vi "test-create-path-trajectory.vi"() -> ()   [LabVIEW 2019]
uses:
  <vilib>/Rock Robotics/WPI/ThirdParty/MJansen/PathPlanner/PathPlanner24.lvlib
  <vilib>/Rock Robotics/WPI/ThirdParty/JAS_Junk/TrajLib/Trajectory_Library.lvlib
  <vilib>/Rock Robotics/WPI/ThirdParty/JAS_Junk/TrajLib/TypeDef/ROTATION2D.ctl
  <vilib>/Rock Robotics/WPI/ThirdParty/JAS_Junk/TrajLib/TypeDef/TRANSLATION2D.ctl
  <vilib>/Rock Robotics/WPI/ThirdParty/JAS_Junk/TrajLib/TypeDef/POSE2D.ctl
  <vilib>/Rock Robotics/WPI/ThirdParty/JAS_Junk/TrajLib/TypeDef/TRAJ_STATE.ctl
  <vilib>/Rock Robotics/WPI/ThirdParty/MJansen/PathPlanner/TypeDef/PathPlannerTrajectoryState.ctl
  <vilib>/Rock Robotics/WPI/ThirdParty/MJansen/PathPlanner/TypeDef/PathPlannerTrajectory.ctl
  <vilib>/Rock Robotics/WPI/ThirdParty/MJansen/PathPlanner/TypeDef/PathPlannerPathConstraints.ctl
  <vilib>/Rock Robotics/WPI/ThirdParty/JAS_Junk/TrajLib/TypeDef/CHASSIS_SPEEDS.ctl
  <vilib>/Rock Robotics/WPI/ThirdParty/MJansen/PathPlanner/TypeDef/PathPlannerGoalEndState.ctl
  <vilib>/Rock Robotics/WPI/ThirdParty/MJansen/PathPlanner/TypeDef/PathPlannerRotationTarget.ctl
  <vilib>/Rock Robotics/WPI/ThirdParty/MJansen/PathPlanner/TypeDef/PathPlannerConstraintsZone.ctl
  <vilib>/Rock Robotics/WPI/ThirdParty/MJansen/PathPlanner/TypeDef/PathPlannerEventMarker.ctl
  <vilib>/Rock Robotics/WPI/ThirdParty/MJansen/PathPlanner/TypeDef/PathPlannerPathPoint.ctl
  <vilib>/Rock Robotics/WPI/ThirdParty/MJansen/PathPlanner/TypeDef/PathPlannerPath.ctl
  <vilib>/Rock Robotics/WPI/ThirdParty/MJansen/PathPlanner/ENum/PathPlanner_CommandUtilType_ENUM.ctl
  <vilib>/Rock Robotics/WPI/ThirdParty/MJansen/PathPlanner/TypeDef/PathPlannerCommandUtil.ctl
  <vilib>/Rock Robotics/WPI/ThirdParty/MJansen/PathPlanner/TypeDef/PathPlannerWaypoint.ctl
  <vilib>/Rock Robotics/WPI/ThirdParty/MJansen/PathPlanner/TypeDef/PathPlannerPointTowardsZone.ctl
  <vilib>/Rock Robotics/WPI/ThirdParty/MJansen/PathPlanner/TypeDef/PathPlannerIdealStartingState.ctl
panel:
  in  "Tab Control":T1(tab)
  in  "Position 1":T2={"TRANSLATION"={"X"=1.0, "Y"=1.0}, "ROTATION"={"VALUE"=0.0, "COS"=1.0, "SIN"=0.0}} {"ROTATION"."SIN" format="%13.4f"; "ROTATION"."COS" format="%13.4f"; "ROTATION"."VALUE" format="%13.4f"; "TRANSLATION"."Y" format="%14.3f"; "TRANSLATION"."X" format="%14.3f"}
  in  "Position 2":T2={"TRANSLATION"={"X"=2.0, "Y"=1.0}, "ROTATION"={"VALUE"=0.0, "COS"=1.0, "SIN"=0.0}} {"ROTATION"."SIN" format="%13.4f"; "ROTATION"."COS" format="%13.4f"; "ROTATION"."VALUE" format="%13.4f"; "TRANSLATION"."Y" format="%14.3f"; "TRANSLATION"."X" format="%14.3f"}
  in  "Position 3":T2={"TRANSLATION"={"X"=3.0, "Y"=1.0}, "ROTATION"={"VALUE"=0.0, "COS"=1.0, "SIN"=0.0}} {"ROTATION"."SIN" format="%13.4f"; "ROTATION"."COS" format="%13.4f"; "ROTATION"."VALUE" format="%13.4f"; "TRANSLATION"."Y" format="%14.3f"; "TRANSLATION"."X" format="%14.3f"}
  in  "Position 4":T2={"TRANSLATION"={"X"=4.0, "Y"=1.0}, "ROTATION"={"VALUE"=0.0, "COS"=1.0, "SIN"=0.0}} {"ROTATION"."SIN" format="%13.4f"; "ROTATION"."COS" format="%13.4f"; "ROTATION"."VALUE" format="%13.4f"; "TRANSLATION"."Y" format="%14.3f"; "TRANSLATION"."X" format="%14.3f"}
  in  "stop":bool
  in  "StartingSpeeds":T5 {"vOmega" format="%10.3f"; "vY" format="%10.3f"; "vX" format="%10.3f"}
  out "Error":bool
  out "Error 2":bool
  out "PathPlannerConstraints":T6={"MaxVelocityMps;"=0.0, "MaxAccelerationMpsSq;"=0.0, "MaxAngularVelRadPsEc;"=0.0, "MaxAngularAccRadPSecSq"=0.0, "Exists"=FALSE, "Unlimited"=FALSE, "NominalVoltageVolts"=12.0}
  out "GoalEndState":T7={"VelocityMPS"=0.0, "Rotation"={"VALUE"=0.0, "COS"=1.0, "SIN"=0.0}} {"Rotation"."SIN" format="%13.4f"; "Rotation"."COS" format="%13.4f"; "Rotation"."VALUE" format="%13.4f"}
  out "PathPlannerPath":T8={"Reversed"=FALSE, "RotationTargets"=[], "ConstraintZones"=[], "EventMarkers"=[], "GlobalConstraints"={"MaxVelocityMps;"=0.0, "MaxAccelerationMpsSq;"=0.0, "MaxAngularVelRadPsEc;"=0.0, "MaxAngularAccRadPSecSq"=0.0, "Exists"=FALSE, "Unlimited"=FALSE, "NominalVoltageVolts"=1.0}, "GoalEndState"={"VelocityMPS"=0.0, "Rotation"={"VALUE"=0.0, "COS"=1.0, "SIN"=0.0}}, "AllPoints"=[], "Name"="", "Waypoints"=[], "PointTowardsZones"=[], "IdealStartingState"={"VelocityMPS"=0.0, "Rotation"={"VALUE"=0.0, "COS"=1.0, "SIN"=0.0}}, "IsChoreoPath"=FALSE, "PreventFlipping"=FALSE} {"IdealStartingState"."Rotation"."SIN" format="%13.4f"; "IdealStartingState"."Rotation"."COS" format="%13.4f"; "IdealStartingState"."Rotation"."VALUE" format="%13.4f"; "PointTowardsZones"."TargetPosition"."Y" format="%14.3f"; "PointTowardsZones"."TargetPosition"."X" format="%14.3f"; "PointTowardsZones"."RotationOffset"."SIN" format="%13.4f"; "PointTowardsZones"."RotationOffset"."COS" format="%13.4f"; "PointTowardsZones"."RotationOffset"."VALUE" format="%13.4f"; "Waypoints"."nextControl"."Y" format="%14.3f"; "Waypoints"."nextControl"."X" format="%14.3f"; "Waypoints"."anchor"."Y" format="%14.3f"; "Waypoints"."anchor"."X" format="%14.3f"; "Waypoints"."prevControl"."Y" format="%14.3f"; "Waypoints"."prevControl"."X" format="%14.3f"; "AllPoints"."RotationTarget"."rotation"."SIN" format="%13.4f"; "AllPoints"."RotationTarget"."rotation"."COS" format="%13.4f"; "AllPoints"."RotationTarget"."rotation"."VALUE" format="%13.4f"; "AllPoints"."Position"."Y" format="%14.3f"; "AllPoints"."Position"."X" format="%14.3f"; "GoalEndState"."Rotation"."SIN" format="%13.4f"; "GoalEndState"."Rotation"."COS" format="%13.4f"; "GoalEndState"."Rotation"."VALUE" format="%13.4f"; "RotationTargets"."rotation"."SIN" format="%13.4f"; "RotationTargets"."rotation"."COS" format="%13.4f"; "RotationTargets"."rotation"."VALUE" format="%13.4f"}
  out "PathPlannerTrajectory":T18 {"States"."TargetHolonomicRotation"."SIN" format="%13.4f"; "States"."TargetHolonomicRotation"."COS" format="%13.4f"; "States"."TargetHolonomicRotation"."VALUE" format="%13.4f"; "States"."Heading"."SIN" format="%13.4f"; "States"."Heading"."COS" format="%13.4f"; "States"."Heading"."VALUE" format="%13.4f"; "States"."PositionMeters"."Y" format="%14.3f"; "States"."PositionMeters"."X" format="%14.3f"}
  out "outPathPlannerStates":T19[](array[typedef]) {"TargetHolonomicRotation"."SIN" format="%13.4f"; "TargetHolonomicRotation"."COS" format="%13.4f"; "TargetHolonomicRotation"."VALUE" format="%13.4f"; "Heading"."SIN" format="%13.4f"; "Heading"."COS" format="%13.4f"; "Heading"."VALUE" format="%13.4f"; "PositionMeters"."Y" format="%14.3f"; "PositionMeters"."X" format="%14.3f"}
  in  "Down Button":bool
  in  "Up Button":bool
  in  "index":i32 step=20
  out "LabVIEWStateCount":i32
  out "LabVIEWStates":T20[](array[typedef]) {"POSE"."ROTATION"."SIN" format="%13.4f"; "POSE"."ROTATION"."COS" format="%13.4f"; "POSE"."ROTATION"."VALUE" format="%13.4f"; "POSE"."TRANSLATION"."Y" format="%14.3f"; "POSE"."TRANSLATION"."X" format="%14.3f"}
  out "XY SPLINE":cluster{dbl[], dbl[]}[](graph)
  out "XY Graph":cluster{dbl[], dbl[]}[](graph)
  out "Sample Graph":dbl[][](graph)
  out "LabVIEW Time Plot":cluster{dbl[], dbl[]}[](graph)
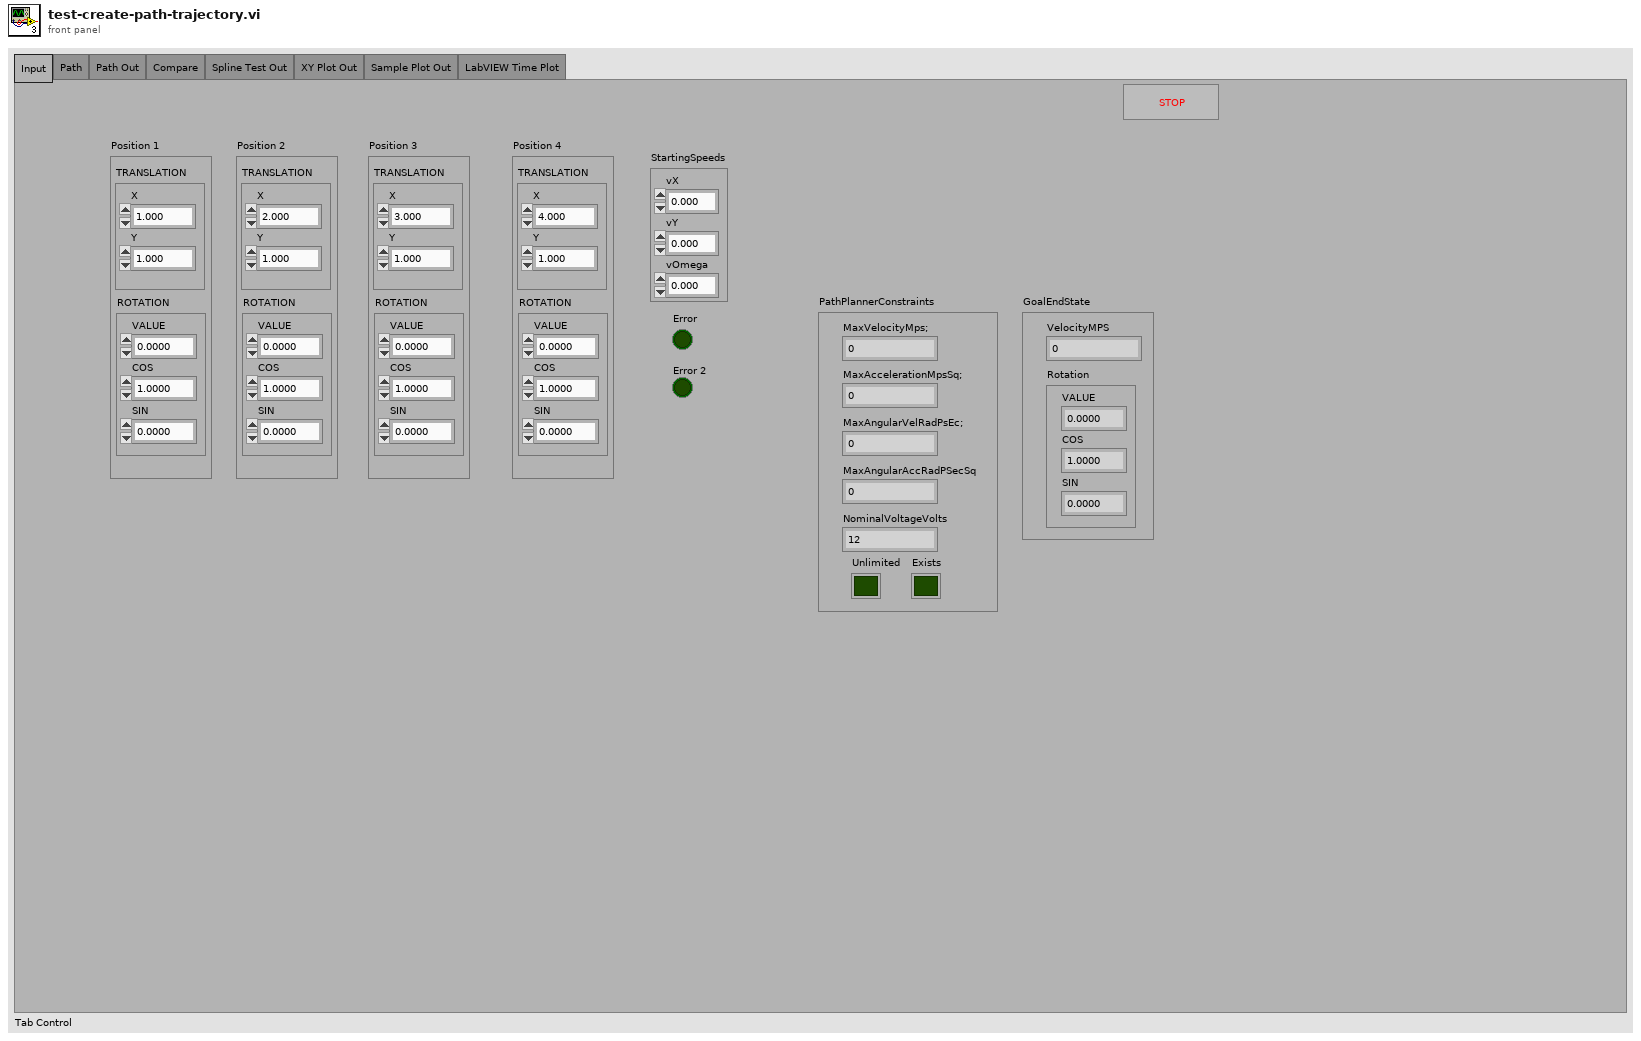
[diagram p1: front panel]
types:
  T1 = enum32{"Input", "Path", "Path Out", "Compare", "Spline Test Out", "XY Plot Out", "Sample Plot Out", "LabVIEW Time Plot"}
  T2 = typedef "Trajectory_Library.lvlib/POSE2D.ctl" = cluster{"TRANSLATION":T3, "ROTATION":T4}
  T3 = typedef "Trajectory_Library.lvlib/TRANSLATION2D.ctl" = cluster{"X":dbl, "Y":dbl}
  T4 = typedef "Trajectory_Library.lvlib/ROTATION2D.ctl" = cluster{"VALUE":dbl, "COS":dbl, "SIN":dbl}
  T5 = typedef "Trajectory_Library.lvlib/CHASSIS_SPEEDS.ctl" = cluster{"vX":dbl, "vY":dbl, "vOmega":dbl}
  T6 = typedef "PathPlanner24.lvlib/PathPlannerPathConstraints.ctl" = cluster{"MaxVelocityMps;":dbl, "MaxAccelerationMpsSq;":dbl, "MaxAngularVelRadPsEc;":dbl, "MaxAngularAccRadPSecSq":dbl, "Exists":bool, "Unlimited":bool, "NominalVoltageVolts":dbl}
  T7 = typedef "PathPlanner24.lvlib/PathPlannerGoalEndState.ctl" = cluster{"VelocityMPS":dbl, "Rotation":T4}
  T8 = typedef "PathPlanner24.lvlib/PathPlannerPath.ctl" = cluster{"Reversed":bool, "RotationTargets":T9[], "ConstraintZones":T10[], "EventMarkers":T11[], "GlobalConstraints":T6, "GoalEndState":T7, "AllPoints":T14[], "Name":string, "Waypoints":T15[], "PointTowardsZones":T16[], "IdealStartingState":T17, "IsChoreoPath":bool, "PreventFlipping":bool}
  T9 = typedef "PathPlanner24.lvlib/PathPlannerRotationTarget.ctl" = cluster{"position":dbl, "rotation":T4, "Exists":bool}
  T10 = typedef "PathPlanner24.lvlib/PathPlannerConstraintsZone.ctl" = cluster{"minPosition":dbl, "maxPosition":dbl, "Constraints":T6, "Present":bool}
  T11 = typedef "PathPlanner24.lvlib/PathPlannerEventMarker.ctl" = cluster{"Position":dbl, "Command":T12, "TriggerName":string, "EndPosition":dbl}
  T12 = typedef "PathPlanner24.lvlib/PathPlannerCommandUtil.ctl" = cluster{"waitTime":dbl, "name":string, "pathName":string, "commands":cluster{"type":T13, "waitTime":dbl, "name":string, "pathName":string}[], "type":T13}
  T13 = typedef "PathPlanner24.lvlib/PathPlanner_CommandUtilType_ENUM.ctl" = enum16{"Unknown", "Wait", "Named", "Path", "Sequential", "Parallel", "Race", "Deadline"}
  T14 = typedef "PathPlanner24.lvlib/PathPlannerPathPoint.ctl" = cluster{"Position":T3, "DistAlongPath":dbl, "MaxV":dbl, "Constraints":T6, "RotationTarget":T9, "WaypointRelativePos":dbl}
  T15 = typedef "PathPlanner24.lvlib/PathPlannerWaypoint.ctl" = cluster{"prevControl":T3, "anchor":T3, "nextControl":T3, "PrevExists":bool, "NextExists":bool}
  T16 = typedef "PathPlanner24.lvlib/PathPlannerPointTowardsZone.ctl" = cluster{"RotationOffset":T4, "Name":string, "TargetPosition":T3, "MinPosition":dbl, "MaxPosition":dbl}
  T17 = typedef "PathPlanner24.lvlib/PathPlannerIdealStartingState.ctl" = cluster{"VelocityMPS":dbl, "Rotation":T4}
  T18 = typedef "PathPlanner24.lvlib/PathPlannerTrajectory.ctl" = cluster{"States":T19[]}
  T19 = typedef "PathPlanner24.lvlib/PathPlannerTrajectoryState.ctl" = cluster{"TimeSeconds":dbl, "VelocityMPS":dbl, "AccerationMpsSq":dbl, "HeadingAngularVelRadPerSec":dbl, "PositionMeters":T3, "Heading":T4, "TargetHolonomicRotation":T4, "CurvatureRadPerMeter":dbl, "PathPlannerConstraints":T6, "DeltaPos":dbl}
  T20 = typedef "Trajectory_Library.lvlib/TRAJ_STATE.ctl" = cluster{"TimeSeconds":dbl, "Velocity":dbl, "Acceleration":dbl, "POSE":T2, "Curvature":dbl}
  T21 = typedef "Trajectory_Library.lvlib/TRAJECTORY.ctl" = cluster{"TotalTImeSecs":dbl, "States":T20[]}
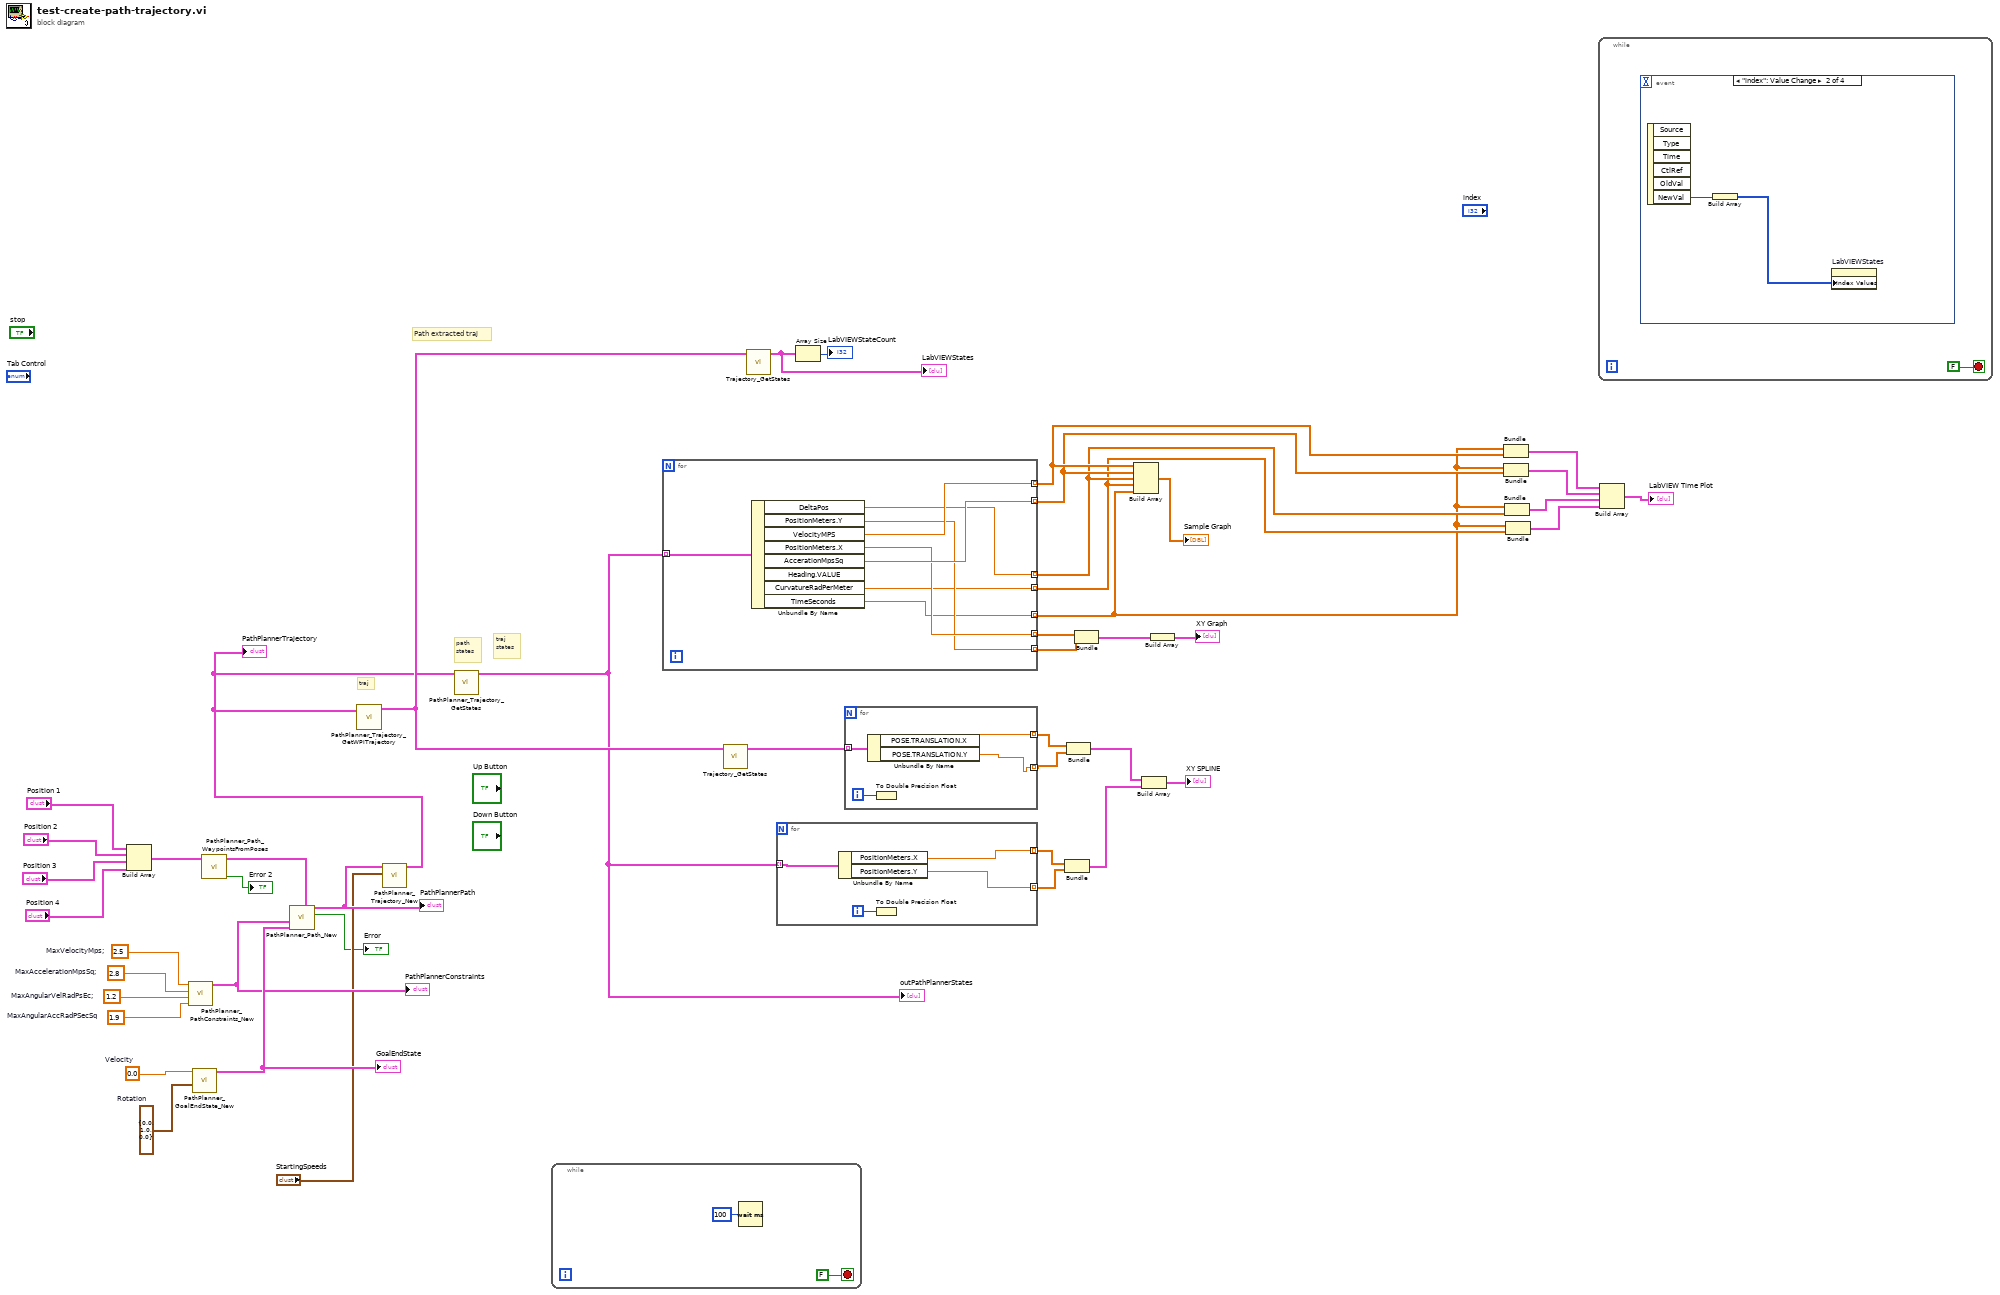
[diagram p0: block diagram]
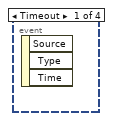
[diagram p2: hidden frame]
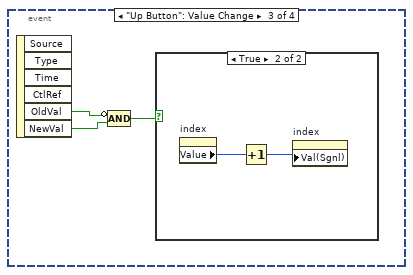
[diagram p3: hidden frame]
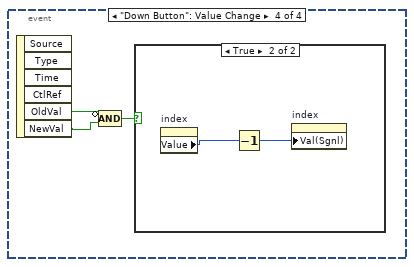
[diagram p5: hidden frame]
diagram:
  w6 = 0.0  # Velocity
  w7 = T4 {"VALUE"=0.0, "COS"=1.0, "SIN"=0.0}  # Rotation
  w9 = 2.5  # MaxVelocityMps;
  w10 = 2.8  # MaxAccelerationMpsSq;
  w11 = 1.2  # MaxAngularVelRadPsEc;
  w8 = 1.9  # MaxAngularAccRadPSecSq
  # "Path extracted traj"
  # "traj"
  # "traj\nstates"
  # "path\nstates"
  n1 = Build Array("Position 1", "Position 2", "Position 3", "Position 4") -> (w15:T2[])
  n2 = call <vilib>:"PathPlanner_PathConstraints_New.vi"("MaxAngularAccRadPSecSq"=w8, "MaxAngularVelRadPsEc;"=w11, "MaxAccelerationMpsSq;"=w10, "MaxVelocityMps;"=w9) -> ("PathPlannerConstraints"=w12:T6)  [unwired: 7 in]
  "PathPlannerConstraints" <- w12
  n3 = call <vilib>:"PathPlanner_GoalEndState_New.vi"("Rotation"=w7, "VelocityMPS"=w6) -> ("GoalEndState"=w13:T7)  [unwired: 9 in]
  "GoalEndState" <- w13
  n4 = call <vilib>:"PathPlanner_Path_WaypointsFromPoses.vi"("Poses"=w15) -> ("Error"=→"Error 2":bool, "Waypoints"=w14:T15[])  [unwired: 9 in]
  n5 = call <vilib>:"PathPlanner_Path_New.vi"("Waypoints"=w14, "GoalEndState"=w13, "GlobalConstraints"=w12) -> ("Error"=→"Error":bool, "PathPlannerPath"=w5:T8)  [unwired: 7 in]
  "PathPlannerPath" <- w5
  n6 = call <vilib>:"PathPlanner_Trajectory_New.vi"("StartingSpeeds"="StartingSpeeds", "Path"=w5) -> ("PathPlannerTrajectory"=w4:T18)  [unwired: 8 in, 1 out]
  "PathPlannerTrajectory" <- w4
  n7 = call <vilib>:"PathPlanner_Trajectory_GetWPITrajectory.vi"("PathPlannerTrajectory"=w4) -> ("WPI TRAJECTORY"=w33:T21)  [unwired: 9 in, 1 out]
  n8 = call <vilib>:"PathPlanner_Trajectory_GetStates.vi"("PathPlannerTrajectory"=w4) -> ("PathPlannerStates"=w30:T19[])  [unwired: 10 in]
  "outPathPlannerStates" <- w30
  n9 = while {
    stop <- FALSE stop-if-true
    n10 = Wait (ms)(milliseconds to wait=u32 100) -> ()  [unwired: 1 out]
  }
  n11 = for {
    tunnel: [w56] -> w28 mode=indexing
    tunnel: [w55] -> w27 mode=indexing
    tunnel: [w50] -> w26 mode=indexing
    tunnel: [w54] -> w45 mode=indexing
    tunnel: [w53] -> w44 mode=indexing
    tunnel: w30 -> [w52] mode=indexing
    tunnel: [w51] -> w25 mode=indexing
    tunnel: [w49] -> w20 mode=indexing
    n12 = Unbundle By Name(w52) -> ("DeltaPos"=w50:dbl, "PositionMeters.Y"=w53:dbl, "VelocityMPS"=w56:dbl, "PositionMeters.X"=w54:dbl, "AccerationMpsSq"=w55:dbl, "CurvatureRadPerMeter"=w51:dbl, "TimeSeconds"=w49:dbl)  [unwired: 1 out]
  }
  n13 = call <vilib>:"Trajectory_GetStates.vi"("TRAJECTORY"=w33) -> ("States"=w34:T20[])  [unwired: 10 in]
  n14 = call <vilib>:"Trajectory_GetStates.vi"("TRAJECTORY"=w33) -> ("States"=w31:T20[])  [unwired: 10 in]
  "LabVIEWStates" <- w31
  n15 = for {
    tunnel: [w59] -> w39 mode=indexing
    tunnel: w30 -> [w58] mode=indexing
    tunnel: [w57] -> w38 mode=indexing
    i -> [w60]
    n16 = Unbundle By Name(w58) -> ("PositionMeters.X"=w59:dbl, "PositionMeters.Y"=w57:dbl)
    n17 = To Double Precision Float(number=w60) -> ()  [unwired: 1 out]
  }
  n18 = Array Size(array=w31) -> (size(s)=→"LabVIEWStateCount":i32)
  n19 = for {
    tunnel: [w63] -> w41 mode=indexing
    tunnel: [w62] -> w40 mode=indexing
    tunnel: w34 -> [w61] mode=indexing
    i -> [w64]
    n20 = Unbundle By Name(w61) -> ("POSE.TRANSLATION.X"=w63:dbl, "POSE.TRANSLATION.Y"=w62:dbl)
    n21 = To Double Precision Float(number=w64) -> ()  [unwired: 1 out]
  }
  n22 = Bundle(w39, w38) -> (w36:cluster{dbl[], dbl[]})  [unwired: 1 in]
  n23 = Bundle(w41, w40) -> (w37:cluster{dbl[], dbl[]})  [unwired: 1 in]
  n24 = Bundle(w45, w44) -> (w43:cluster{dbl[], dbl[]})  [unwired: 1 in]
  n25 = Build Array(w28, w27, w26, w25, w20) -> (→"Sample Graph":dbl[][])
  n26 = Build Array(w37, w36) -> (→"XY SPLINE":cluster{dbl[], dbl[]}[])
  n27 = Build Array(w43) -> (→"XY Graph":cluster{dbl[], dbl[]}[])
  n28 = Bundle(w20, w28) -> (w24:cluster{dbl[], dbl[]})  [unwired: 1 in]
  n29 = Bundle(w20, w27) -> (w23:cluster{dbl[], dbl[]})  [unwired: 1 in]
  n30 = Bundle(w20, w26) -> (w22:cluster{dbl[], dbl[]})  [unwired: 1 in]
  n31 = Bundle(w20, w25) -> (w21:cluster{dbl[], dbl[]})  [unwired: 1 in]
  n32 = while {
    stop <- FALSE stop-if-true
    n33 = event shown="[1] \"index\": Value Change" {
      selector: _ -> [_ _ _ _]
      dyn-events: _ -> [_ _ _ _]
      timeout: _ -> [_ _ _ _]
      event Timeout {
        n34 = event-data() -> ()  [unwired: 1 in, 3 out]
      }
      event "index": Value Change {
        n35 = event-data() -> ("NewVal"=w67:i32)  [unwired: 1 in, 5 out]
        n36 = Build Array(w67) -> (w66:i32[])
        n37 = property on="LabVIEWStates" class="Arr (strict)"("Index Values"=w66) -> ()  [unwired: 2 in, 2 out]
      }
      event "Up Button": Value Change {
        n38 = event-data() -> ("OldVal"=w70:bool, "NewVal"=w69:bool)  [unwired: 1 in, 4 out]
        n39 = Compound Arithmetic op=AND(invert w70, w69) -> (w68:bool)
        n40 = case shown="True" w68 {
          frame False {
          }
          frame True {
            n41 = property on="index" class="DigNum (strict)"() -> ("Value"=w71:i32)  [unwired: 2 in, 2 out]
            n42 = Increment(x=w71) -> (x+1=w72:i32)
            n43 = property on="index" class="DigNum (strict)"("Val(Sgnl)"=w72) -> ()  [unwired: 2 in, 2 out]
          }
        }
      }
      event "Down Button": Value Change {
        n44 = event-data() -> ("OldVal"=w74:bool, "NewVal"=w73:bool)  [unwired: 1 in, 4 out]
        n45 = Compound Arithmetic op=AND(invert w74, w73) -> (w75:bool)
        n46 = case shown="True" w75 {
          frame False {
          }
          frame True {
            n47 = property on="index" class="DigNum (strict)"() -> ("Value"=w76:i32)  [unwired: 2 in, 2 out]
            n48 = Decrement(x=w76) -> (x-1=w77:i32)
            n49 = property on="index" class="DigNum (strict)"("Val(Sgnl)"=w77) -> ()  [unwired: 2 in, 2 out]
          }
        }
      }
    }
  }
  n50 = Build Array(w24, w23, w22, w21) -> (→"LabVIEW Time Plot":cluster{dbl[], dbl[]}[])
